vi "Mass Flow Meters.vi"(11 "Array in":dbl[](array[numeric])) -> (3 "Array out":dbl[](array[numeric]))   [LabVIEW 2017]
uses:
  <vilib>/ptbypt/NI_PtbyPt.lvlib
panel:
  out "AI7":dbl
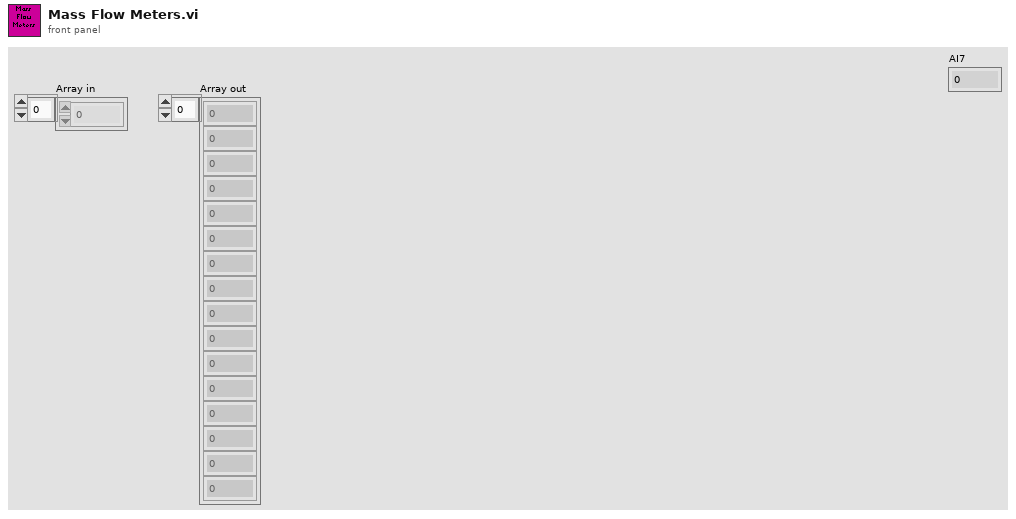
[diagram p1: front panel]
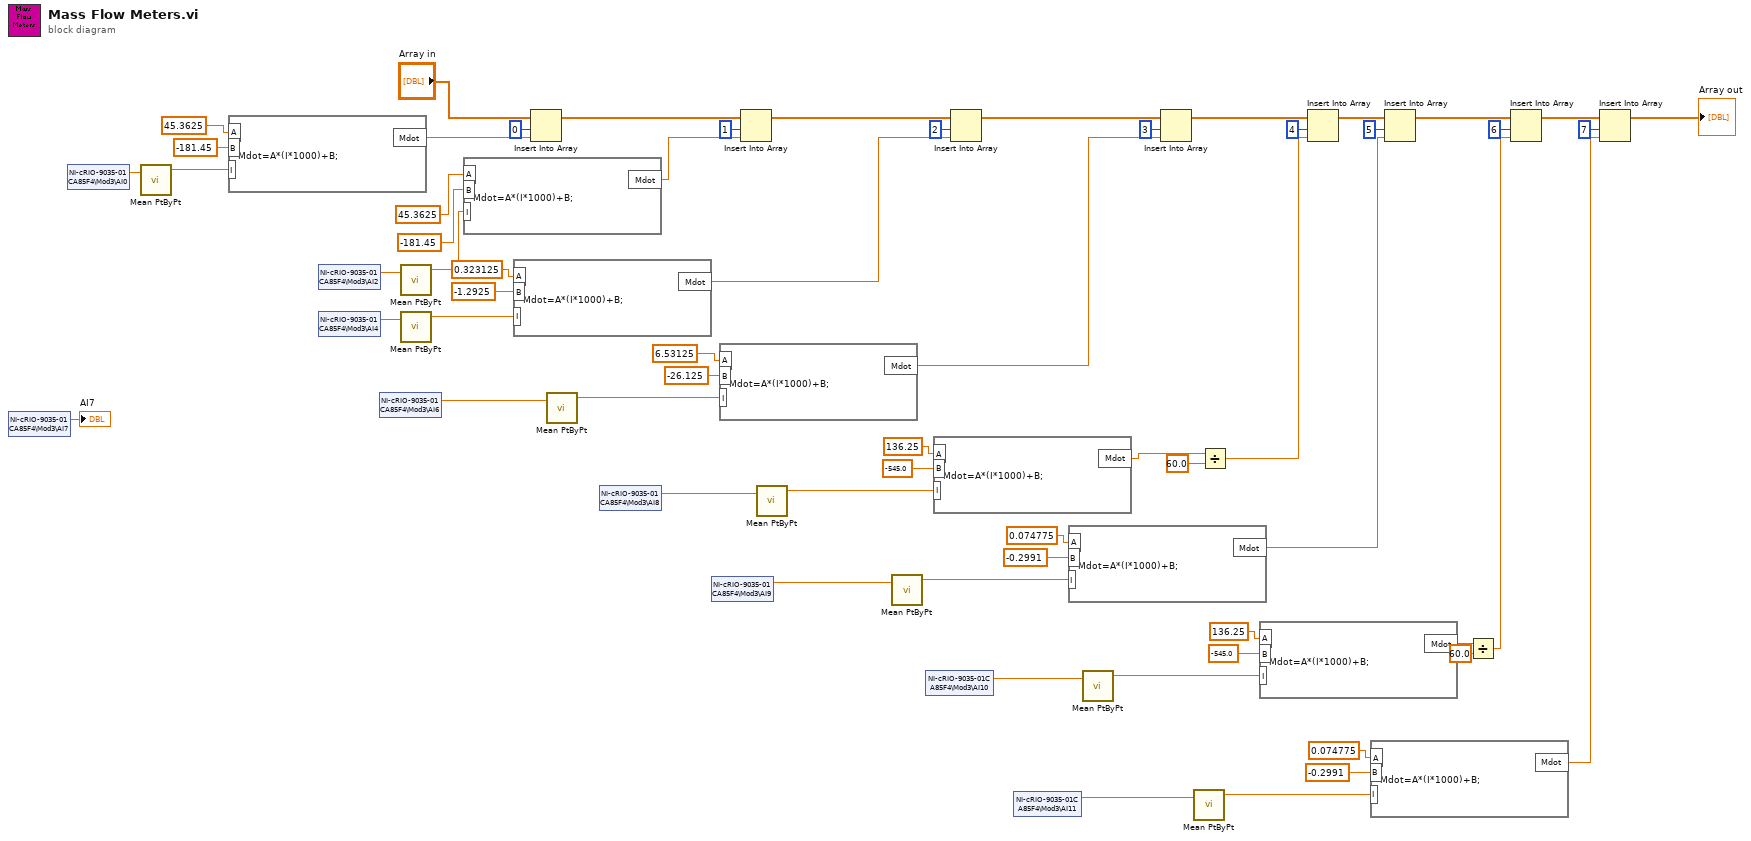
[diagram p0: block diagram]
diagram:
  n1 = shared-variable "NI-cRIO-9035-01CA85F4\\Mod3\\AI7"() -> (→"AI7":dbl)  [unwired: 1 in, 1 out]
  n2 = shared-variable "NI-cRIO-9035-01CA85F4\\Mod3\\AI0"() -> (w36:dbl)  [unwired: 1 in, 1 out]
  n3 = call <vilib>:"Mean PtByPt.vi"("x"=w36) -> ("mean"=w35:dbl)  [unwired: 3 in, 1 out]
  n4 = formula code="Mdot=A*(I*1000)+B;"("I"=w35, "A"=45.3625 ("input variable"), "B"=-181.45 ("input variable")) -> ("Mdot"=w38:dbl)
  n5 = shared-variable "NI-cRIO-9035-01CA85F4\\Mod3\\AI2"() -> (w62:dbl)  [unwired: 1 in, 1 out]
  n6 = shared-variable "NI-cRIO-9035-01CA85F4\\Mod3\\AI4"() -> (w61:dbl)  [unwired: 1 in, 1 out]
  n7 = shared-variable "NI-cRIO-9035-01CA85F4\\Mod3\\AI6"() -> (w60:dbl)  [unwired: 1 in, 1 out]
  n8 = call <vilib>:"Mean PtByPt.vi"("x"=w62) -> ("mean"=w41:dbl)  [unwired: 3 in, 1 out]
  n9 = call <vilib>:"Mean PtByPt.vi"("x"=w61) -> ("mean"=w44:dbl)  [unwired: 3 in, 1 out]
  n10 = formula code="Mdot=A*(I*1000)+B;"("I"=w41, "A"=45.3625 ("input variable"), "B"=-181.45 ("input variable")) -> ("Mdot"=w32:dbl)
  n11 = formula code="Mdot=A*(I*1000)+B;"("I"=w44, "A"=0.323125 ("input variable"), "B"=-1.2925 ("input variable")) -> ("Mdot"=w31:dbl)
  n12 = Insert Into Array(array="Array in", index=0, new element=w38) -> (w54:dbl[])
  n13 = call <vilib>:"Mean PtByPt.vi"("x"=w60) -> ("mean"=w47:dbl)  [unwired: 3 in, 1 out]
  n14 = shared-variable "NI-cRIO-9035-01CA85F4\\Mod3\\AI8"() -> (w59:dbl)  [unwired: 1 in, 1 out]
  n15 = shared-variable "NI-cRIO-9035-01CA85F4\\Mod3\\AI9"() -> (w19:dbl)  [unwired: 1 in, 1 out]
  n16 = formula code="Mdot=A*(I*1000)+B;"("I"=w47, "A"=6.53125 ("input variable"), "B"=-26.125 ("input variable")) -> ("Mdot"=w30:dbl)
  n17 = Insert Into Array(array=w54, index=1, new element=w32) -> (w55:dbl[])
  n18 = call <vilib>:"Mean PtByPt.vi"("x"=w59) -> ("mean"=w50:dbl)  [unwired: 3 in, 1 out]
  n19 = call <vilib>:"Mean PtByPt.vi"("x"=w19) -> ("mean"=w22:dbl)  [unwired: 3 in, 1 out]
  n20 = shared-variable "NI-cRIO-9035-01CA85F4\\Mod3\\AI10"() -> (w58:dbl)  [unwired: 1 in, 1 out]
  n21 = formula code="Mdot=A*(I*1000)+B;"("I"=w50, "A"=136.25 ("input variable"), "B"=-545.0 ("input variable")) -> ("Mdot"=w6:dbl)
  n22 = Insert Into Array(array=w55, index=2, new element=w31) -> (w56:dbl[])
  n23 = shared-variable "NI-cRIO-9035-01CA85F4\\Mod3\\AI11"() -> (w11:dbl)  [unwired: 1 in, 1 out]
  n24 = formula code="Mdot=A*(I*1000)+B;"("I"=w22, "A"=0.074775 ("input variable"), "B"=-0.2991 ("input variable")) -> ("Mdot"=w18:dbl)
  n25 = call <vilib>:"Mean PtByPt.vi"("x"=w58) -> ("mean"=w53:dbl)  [unwired: 3 in, 1 out]
  n26 = Insert Into Array(array=w56, index=3, new element=w30) -> (w57:dbl[])
  n27 = call <vilib>:"Mean PtByPt.vi"("x"=w11) -> ("mean"=w14:dbl)  [unwired: 3 in, 1 out]
  n28 = Divide(x=w6, y=60.0) -> (x/y=w4:dbl)
  n29 = formula code="Mdot=A*(I*1000)+B;"("I"=w53, "A"=136.25 ("input variable"), "B"=-545.0 ("input variable")) -> ("Mdot"=w3:dbl)
  n30 = Insert Into Array(array=w57, index=4, new element=w4) -> (w16:dbl[])
  n31 = formula code="Mdot=A*(I*1000)+B;"("I"=w14, "A"=0.074775 ("input variable"), "B"=-0.2991 ("input variable")) -> ("Mdot"=w9:dbl)
  n32 = Insert Into Array(array=w16, index=5, new element=w18) -> (w15:dbl[])
  n33 = Divide(x=w3, y=60.0) -> (x/y=w1:dbl)
  n34 = Insert Into Array(array=w15, index=6, new element=w1) -> (w10:dbl[])
  n35 = Insert Into Array(array=w10, index=7, new element=w9) -> (→"Array out":dbl[])
